vi "WebDAV_Get_Files.vi"() -> ()   [LabVIEW 2014]
uses:
  <vilib>/WebDAVClient/Simple Get File.vi
  <vilib>/WebDAVClient/NI_WebDAV.lvlib
panel:
  in  "directory/filename":string="get.txt"
  in  "remote file uri":string="ftp://169.254.254.10/ni-rt/startup/sample/sample3.txt"
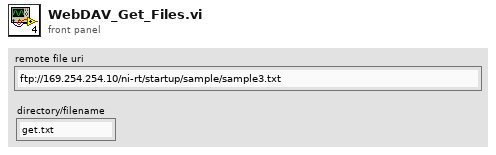
[diagram p1: front panel]
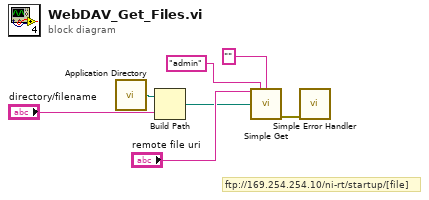
[diagram p0: block diagram]
diagram:
  # "ftp://169.254.254.10/ni-rt/startup/[file]"
  n1 = call <vilib>:"Application Directory.vi"() -> ("Application Directory"=w6:path)
  n2 = Build Path(base path=w6, name or relative path="directory/filename") -> (appended path=w5:path)
  n3 = call-poly <vilib>:"Simple Get.vi"("remote file uri"="remote file uri", "username"="admin", "password"="", "local file path"=w5) -> ("error out"=w1:errorcluster)  [unwired: 10 in, 1 out]
  n4 = call <vilib>:"Simple Error Handler.vi"("error in (no error)"=w1) -> ()  [unwired: 4 in, 5 out]
